vi "build-filepath.vi"(4 "Include Seconds in Filename":bool, 6 "Include Time in Filename":bool=TRUE, 7 "Log Filepath Source":T1(ring), 8 "Include Date in Filename":bool=TRUE, 9 "log file name":string="log", 10 "Log File Folder Name":string="log", 11 "Log File Path":path=path "C:/Users/dheard/Documents/0002-labview-projects/ammonia-absorbsion-rig/data") -> (3 "appended path for log file":path, 5 "date string":string)   [LabVIEW 2023]
panel:
  out "Application Directory":path
  out "datetime-mode":u32
  out "log folder path":path
  out "stripped path":path
  out "vi path":path
  # "Filepath"
  # "Select Auto/Manual Log Filepath"
  # "Manual Selection"
  # "File Name"
  # "Auto Generation"
  # "Path is relative to application or VI"
  # "Path Stripped to Local Directory"
  # "Select or Create Subdirectory with this name"
  # "Name Log File"
  # "This will be the path log files are saved to"
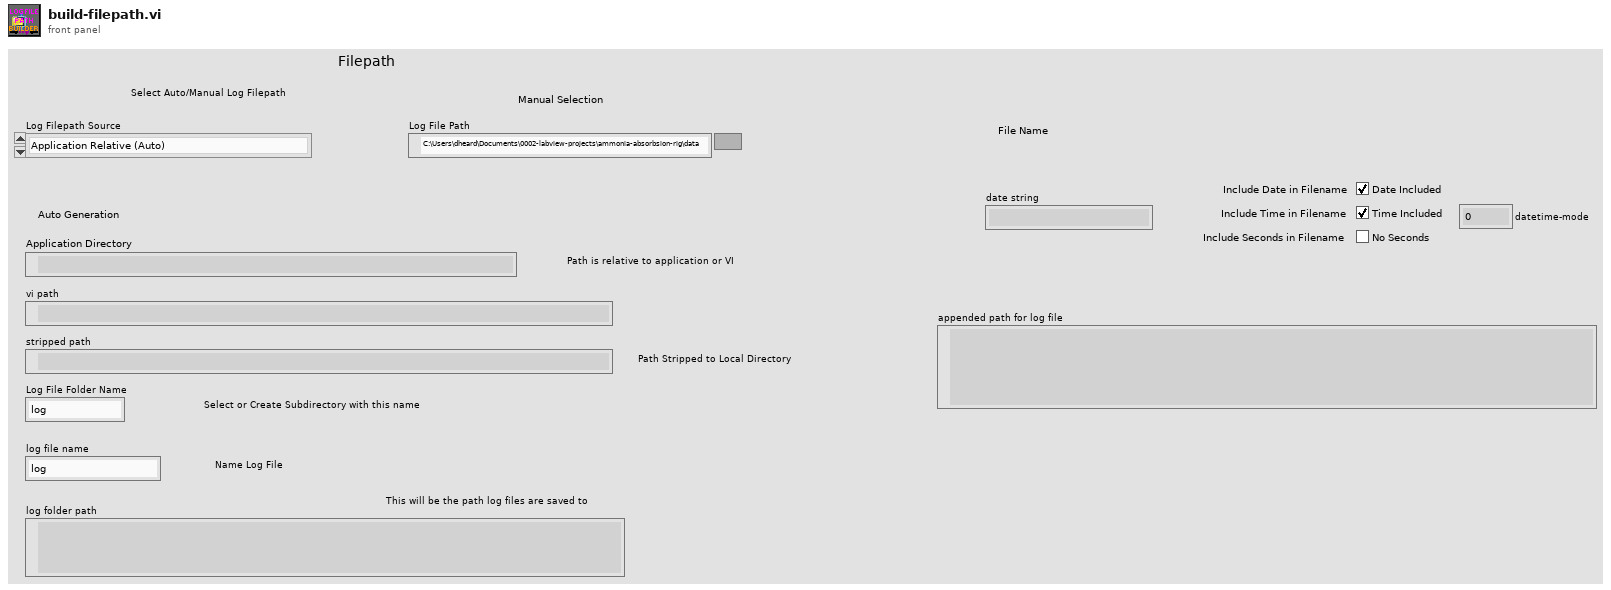
[diagram p1: front panel]
types:
  T1 = enum16{"Application Relative (Auto)", "VI Relative (Auto)", "Complete Path (Manual)"}
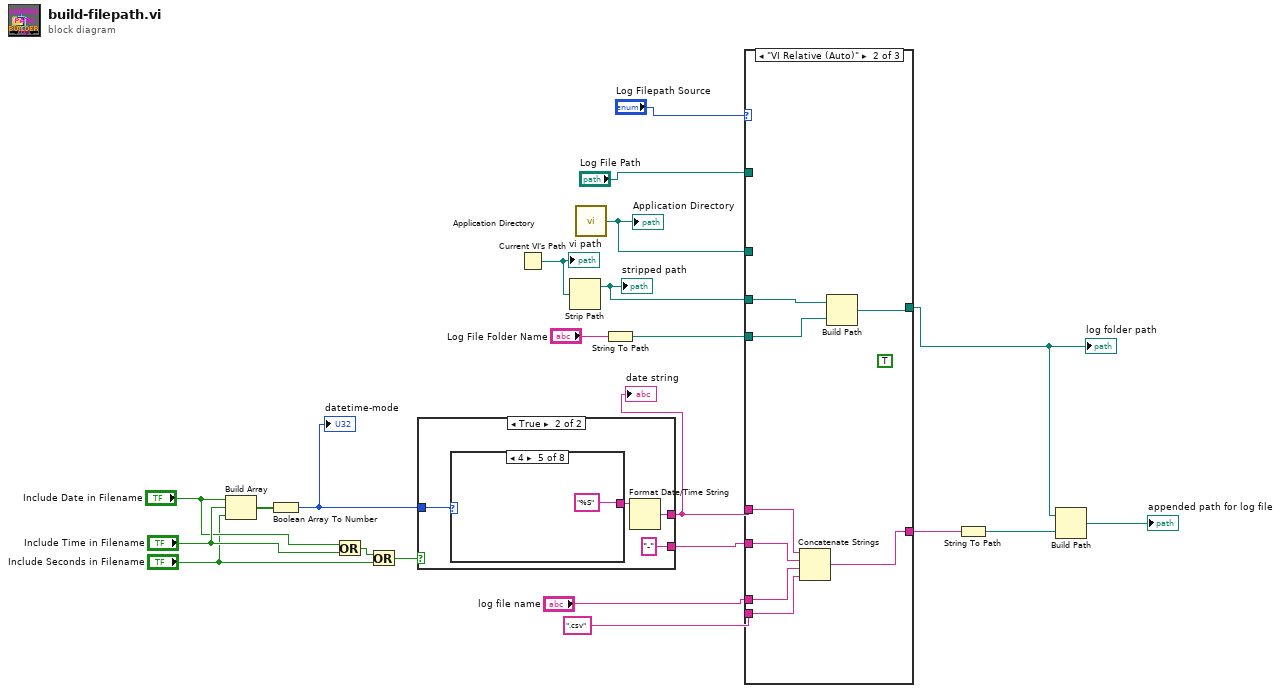
[diagram p0: block diagram]
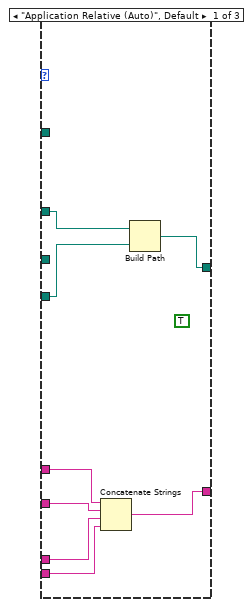
[diagram p2: hidden frame]
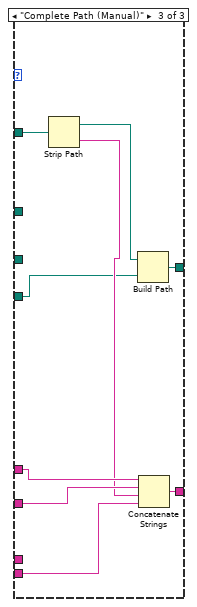
[diagram p3: hidden frame]
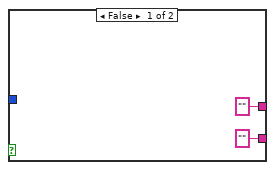
[diagram p4: hidden frame]
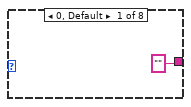
[diagram p5: hidden frame]
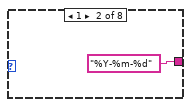
[diagram p6: hidden frame]
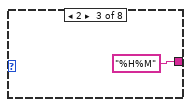
[diagram p7: hidden frame]
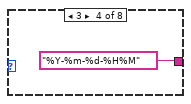
[diagram p8: hidden frame]
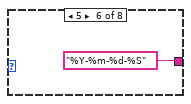
[diagram p9: hidden frame]
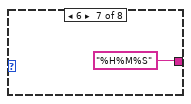
[diagram p10: hidden frame]
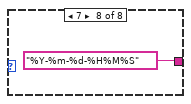
[diagram p11: hidden frame]
diagram:
  n1 = Build Array("Include Date in Filename", "Include Time in Filename", "Include Seconds in Filename") -> (w16:bool[])
  n2 = Boolean Array To Number(Boolean array=w16) -> (number=w22:u32)
  "datetime-mode" <- w22
  n3 = Or(x="Include Date in Filename", y="Include Time in Filename") -> (x .or. y?=w17:bool)
  n4 = Or(x=w17, y="Include Seconds in Filename") -> (x .or. y?=w18:bool)
  n5 = case shown="True" w18 {
    tunnel: ["" ("date/time string") w28] -> w6
    tunnel: w22 -> [_ w26]
    tunnel: ["" ("string") "-" ("string")] -> w5
    frame False {
    }
    frame True {
      n6 = case shown="4" w26 {
        tunnel: ["" ("time format string (%c)") "%Y-%m-%d" ("time format string (%c)") "%H%M" ("time format string (%c)") "%Y-%m-%d-%H%M" ("time format string (%c)") "%S" ("time format string (%c)") "%Y-%m-%d-%S" ("time format string (%c)") "%H%M%S" ("time format string (%c)") "%Y-%m-%d-%H%M%S" ("time format string (%c)")] -> w27
        frame 0, Default {
        }
        frame 1 {
        }
        frame 2 {
        }
        frame 3 {
        }
        frame 4 {
        }
        frame 5 {
        }
        frame 6 {
        }
        frame 7 {
        }
      }
      n7 = Format Date/Time String(time format string (%c)=w27) -> (date/time string=w28:string)  [unwired: 2 in]
    }
  }
  "date string" <- w6
  n8 = Current VI's Path() -> (path=w13:path)
  "vi path" <- w13
  n9 = Strip Path(path=w13) -> (stripped path=w12:path)  [unwired: 1 out]
  "stripped path" <- w12
  n10 = call <vilib>:"Application Directory.vi"() -> ("Application Directory"=w11:path)
  "Application Directory" <- w11
  n11 = String To Path(string="Log File Folder Name") -> (path=w7:path)
  n12 = case shown="\"VI Relative (Auto)\"" "Log Filepath Source" {
    tunnel: w12 -> [_ w47 _]
    tunnel: w11 -> [w39 _ _]
    tunnel: "Log File Path" -> [_ _ w57]
    tunnel: w7 -> [w37 w46 w55]
    tunnel: w6 -> [w41 w51 w59]
    tunnel: w5 -> [w42 w50 w61]
    tunnel: "log file name" -> [w44 w49 _]
    tunnel: ".csv" ("string") -> [w43 w48 w58]
    tunnel: [w40 w52 w60] -> w2
    tunnel: [w38 w45 w53] -> w1
    frame "Application Relative (Auto)", Default {
      (unwired) TRUE
      n13 = Concatenate Strings(w41, w42, w44, w43) -> (w40:string)
      n14 = Build Path(base path=w39, name or relative path=w37) -> (appended path=w38:path)
    }
    frame "VI Relative (Auto)" {
      (unwired) TRUE
      n15 = Concatenate Strings(w51, w50, w49, w48) -> (w52:string)
      n16 = Build Path(base path=w47, name or relative path=w46) -> (appended path=w45:path)
    }
    frame "Complete Path (Manual)" {
      n17 = Strip Path(path=w57) -> (stripped path=w54:path, name=w56:string)
      n18 = Build Path(base path=w54, name or relative path=w55) -> (appended path=w53:path)
      n19 = Concatenate Strings(w59, w61, w56, w58) -> (w60:string)
    }
  }
  "log folder path" <- w1
  n20 = String To Path(string=w2) -> (path=w15:path)
  n21 = Build Path(base path=w1, name or relative path=w15) -> (appended path=→"appended path for log file":path)
